vi "Data Buffer Test Program subvi.vi"(9 "millisecond multiple":u32=1000, 10 "Mult":dbl=1.0, 11 "Data Buffer in":refnum<class "Data Buffer.lvclass">) -> ()   [LabVIEW 2022 SP3]
uses:
  Data Buffer.lvclass
panel:
  out "error out":errorcluster
  out "XY Graph":T1(graph)
  in  "stop":bool
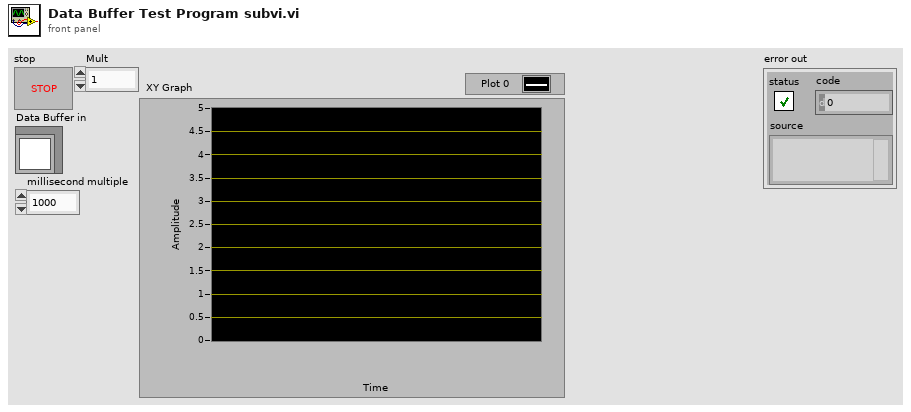
[diagram p1: front panel]
types:
  T1 = cluster{cluster{"Time Stamp":timestamp, "Numeric":dbl}[]}[]
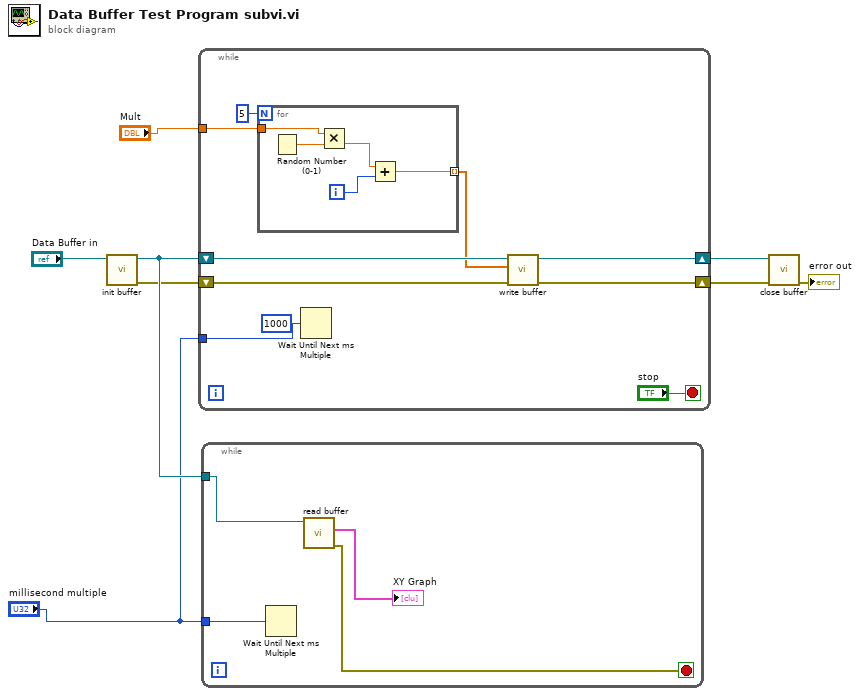
[diagram p0: block diagram]
diagram:
  n1 = call-dynamic "init buffer.vi"("Data Buffer in"="Data Buffer in") -> ("error out"=w6:errorcluster, "Data Buffer out"=w7:refnum<class "Data Buffer.lvclass">)  [unwired: 9 in]
  n2 = while {
    shift-right: [w13] -> w8
    shift-left: w7 -> [w15]
    shift-right: [w11] -> w5
    shift-left: w6 -> [w12]
    tunnel: "Mult" -> [w10]
    tunnel: "millisecond multiple" -> [w9]
    stop <- "stop" stop-if-true
    (unwired) u32 1000 ("millisecond multiple")
    n3 = for {
      N: 5 -> [_]
      tunnel: [w20] -> w14 mode=indexing
      tunnel: w10 -> [w18]
      i -> [w21]
      n4 = Random Number (0-1)() -> (number: 0 to 1=w22:dbl)
      n5 = Multiply(x=w18, y=w22) -> (x*y=w19:dbl)
      n6 = Add(x=w19, y=w21) -> (x+y=w20:dbl)
    }
    n7 = Wait Until Next ms Multiple(millisecond multiple=w9) -> ()  [unwired: 1 out]
    n8 = call-dynamic "write buffer.vi"("error in (no error)"=w12, "Data"=w14, "Data Buffer in"=w15) -> ("error out"=w11:errorcluster, "Data Buffer out"=w13:refnum<class "Data Buffer.lvclass">)  [unwired: 7 in]
  }
  n9 = while {
    tunnel: w7 -> [w26]
    tunnel: "millisecond multiple" -> [w23]
    stop <- w24 stop-if-true
    n10 = Wait Until Next ms Multiple(millisecond multiple=w23) -> ()  [unwired: 1 out]
    n11 = call-dynamic "read buffer.vi"("Data Buffer in"=w26) -> ("error out"=w24:errorcluster, "XY Graph"=→"XY Graph":T1)  [unwired: 8 in, 1 out]
  }
  n12 = call-dynamic "close buffer.vi"("error in (no error)"=w5, "Data Buffer in"=w8) -> ("error out"=→"error out":errorcluster)  [unwired: 8 in, 1 out]
